vi "231124_Cluster_MAJ.vi"(8 "error in (no error)":errorcluster, 9 "Nikon status cluster":T2, 10 "Cluster commandes":T1={"Dia lamp"=TRUE, "Dia lamp intensity"=1689.1304347826087, "Objective"=2, "Light path"=2, "Z pos (µm)"=335593} {"Z pos (µm)" min=0 max=990000 step=100 scale=0.0..990000.0; "Light path" items=["1- Eyepiece"=1, "2- Right"=2, "3- Left + Eyepiece"=3, "4- Left"=4]; "Objective" items=["1- Target"=1, "2- PLAN APO 100X 1,45 Oil"=2, "3- Empty"=3, "4- Empty"=4, "5- Empty"=5, "6- Empty"=6]; "Dia lamp intensity" scale=0.0..2100.0}, 11 "Cluster commandes":refnum<vi>) -> (0 "error out":errorcluster, 2 "Cluster out":T1={"Dia lamp"=TRUE, "Dia lamp intensity"=1689.1304347826087, "Objective"=2, "Light path"=2, "Z pos (µm)"=335593} {"Z pos (µm)" min=0 max=990000 step=100 scale=0.0..990000.0; "Light path" items=["1- Eyepiece"=1, "2- Right"=2, "3- Left + Eyepiece"=3, "4- Left"=4]; "Objective" items=["1- Target"=1, "2- PLAN APO 100X 1,45 Oil"=2, "3- Empty"=3, "4- Empty"=4, "5- Empty"=5, "6- Empty"=6]; "Dia lamp intensity" scale=0.0..2100.0}, 3 "iLIGHTPATH":i32)   [LabVIEW 2024]
doc: "This vi updates the microscope status cluster.\nThe output is the status of the lightpath (to further display green LEDs accordingly"
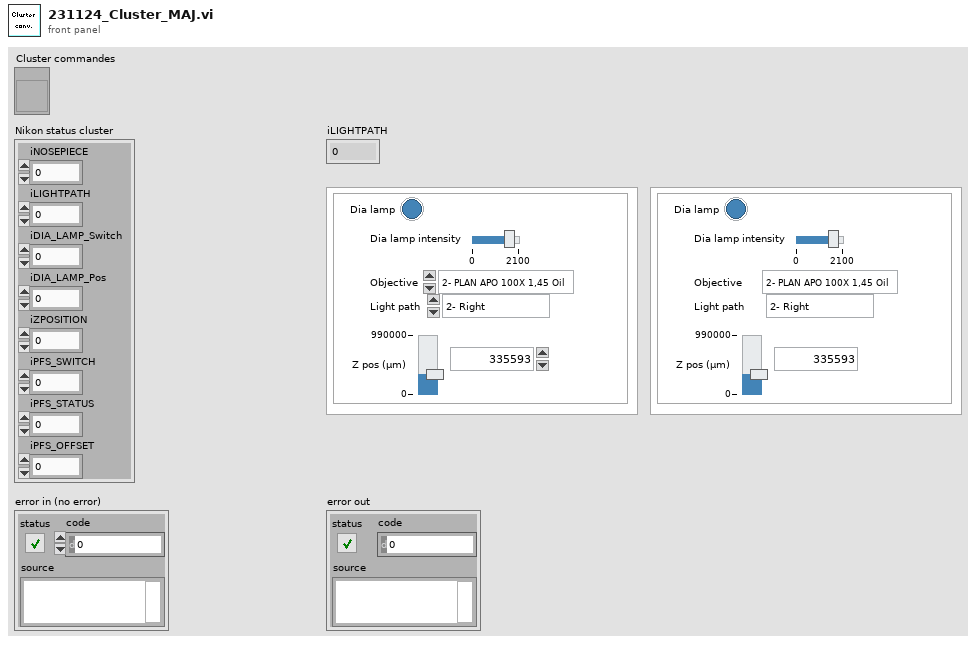
[diagram p1: front panel]
types:
  T1 = cluster{"Dia lamp":bool, "Dia lamp intensity":dbl, "Objective":i32, "Light path":u32, "Z pos (µm)":i32}
  T2 = cluster{"iNOSEPIECE":i32, "iLIGHTPATH":i32, "iDIA_LAMP_Switch":i32, "iDIA_LAMP_Pos":i32, "iZPOSITION":i32, "iPFS_SWITCH":i32, "iPFS_STATUS":i32, "iPFS_OFFSET":i32}
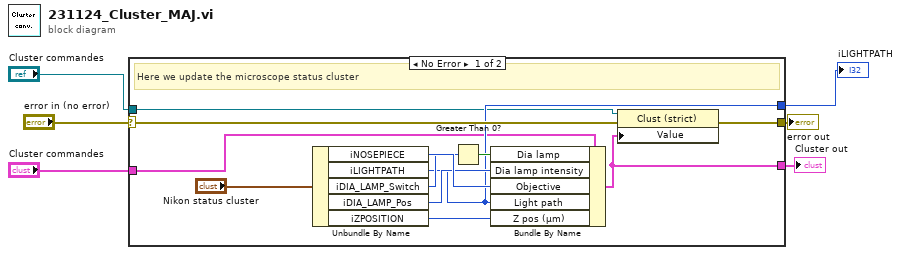
[diagram p0: block diagram]
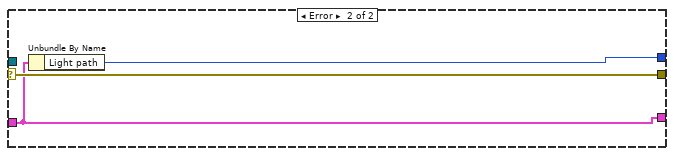
[diagram p2: hidden frame]
diagram:
  n1 = case shown="No Error" "error in (no error)" {
    selector: "error in (no error)" -> [w11 w21]
    tunnel: [w12 w21] -> w6
    tunnel: [w10 w20] -> w4
    tunnel: "Cluster commandes" -> [w9 w19]
    tunnel: "Cluster commandes" -> [w8 _]
    tunnel: [w7 w19] -> w1
    frame No Error {
      # "Here we update the microscope status cluster"
      n2 = Unbundle By Name("Nikon status cluster") -> ("iNOSEPIECE"=w17:i32, "iLIGHTPATH"=w10:i32, "iDIA_LAMP_Switch"=w14:i32, "iDIA_LAMP_Pos"=w15:i32, "iZPOSITION"=w18:i32)
      n3 = Greater Than 0?(x=w14) -> (x > 0?=w16:bool)
      n4 = Bundle By Name(cluster=w9, "Dia lamp"=w16, "Dia lamp intensity"=w15, "Objective"=w17, "Light path"=w10, "Z pos (µm)"=w18) -> (w7:T1)
      n5 = property on="Property Node" class="Clust (strict)"(reference=w8, error in=w11, "Value"=w7) -> (error out=w12:errorcluster)  [unwired: 1 out]
    }
    frame Error {
      n6 = Unbundle By Name(w19) -> ("Light path"=w20:u32)
    }
  }
  "error out" <- w6
  "iLIGHTPATH" <- w4
  "Cluster out" <- w1
